vi "DumbDash Control Filter.vi"(11 "Ctl Refnum":refnum<vi>) -> (2 "Keep?":bool)   [LabVIEW 2014]
uses:
  DumbDash Control Type.ctl
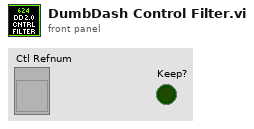
[diagram p1: front panel]
types:
  T1 = typedef "DumbDash Control Type.ctl" = enum16{"Invalid", "Number", "Boolean", "String"}
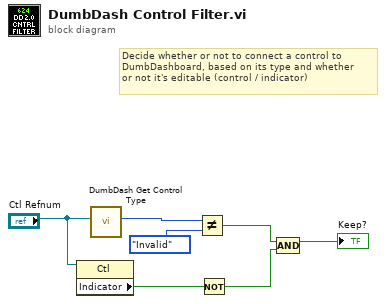
[diagram p0: block diagram]
diagram:
  # "Decide whether or not to connect a control to\nDumbDashboard, based on its type and whether\nor not it's editable (control / indicator)"
  n1 = property class="Ctl"(reference="Ctl Refnum") -> ("Indicator"=w4:bool)  [unwired: 1 in, 2 out]
  n2 = call "DumbDash Get Control Type.vi"("reference"="Ctl Refnum") -> ("Type"=w7:T1)  [unwired: 10 in]
  n3 = Not Equal?(x=w7, y=DumbDash_Control_Type."Invalid") -> (x != y?=w3:bool)
  n4 = Not(x=w4) -> (.not. x?=w2:bool)
  n5 = Compound Arithmetic op=AND(w3, w2) -> (→"Keep?":bool)
